vi "LV FPGA Serial Read Write.vi"(0 "Transmit":refnum<k21>="Port8/DIO0", 1 "Read FIFO":refnum<k21>="Read FIFO", 2 "Write FIFO":refnum<k21>="Write FIFO", 5 "Receive":refnum<k21>="Port8/DIOCTL", 7 "baud rate (9600)":u32=9600, 9 "data bits (8)":i32=8 min=5 max=8 step=1, 11 "parity (0:none)":enum16{"None", "Odd", "Even", "Mark", "Space"}(ring), 12 "stop bits (10: 1 bit)":u16(ring)=10 items=["1.0"=10, "1.5"=15, "2.0"=20], 13 "Invert Polarity?":bool) -> ()   [LabVIEW 2010]
panel:
  out "Read: Transmission Error":bool
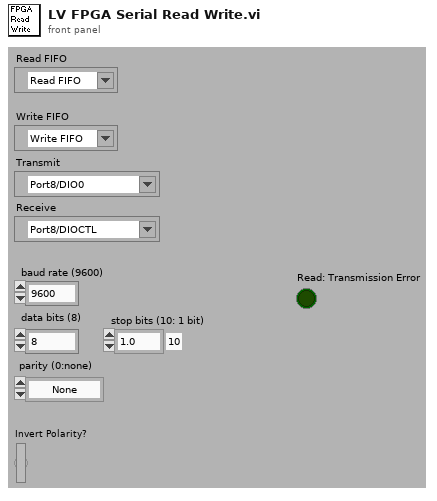
[diagram p1: front panel]
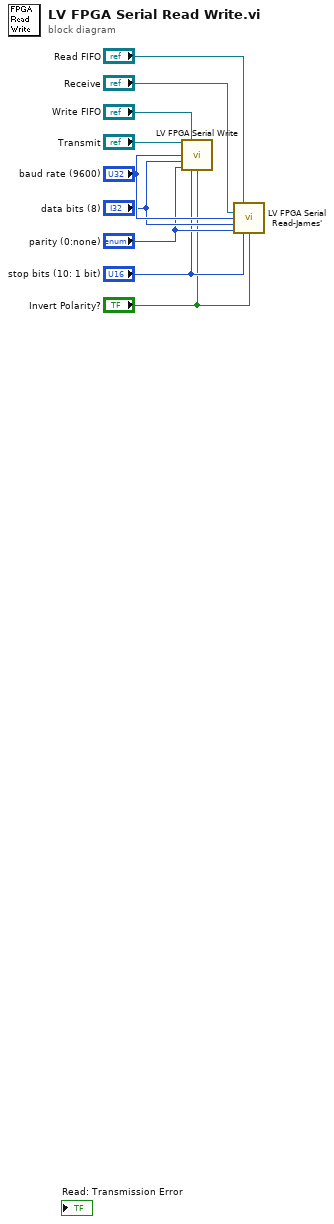
[diagram p0: block diagram]
diagram:
  n1 = call "LV FPGA Serial Write.vi"("Transmit"="Transmit", "Write FIFO"="Write FIFO", "baud rate (9600)"="baud rate (9600)", "data bits (8)"="data bits (8)", "parity (0:none)"="parity (0:none)", "stop bits (10: 1 bit)"="stop bits (10: 1 bit)", "Invert Polarity?"="Invert Polarity?") -> ()  [unwired: 9 in]
  n2 = call "LV FPGA Serial Read-James'.vi"("Read FIFO"="Read FIFO", "Receive"="Receive", "baud rate (9600)"="baud rate (9600)", "data bits (8)"="data bits (8)", "parity (0:none)"="parity (0:none)", "stop bits (10: 1 bit)"="stop bits (10: 1 bit)", "Invert Polarity?"="Invert Polarity?") -> ()  [unwired: 9 in]
